vi "Execute Menu Action.vi"(8 "error in":errorcluster, 10 "Item Tag":string, 11 "Peer Review in":refnum<class "Peer Review.lvclass">) -> (0 "error out":errorcluster, 3 "Peer Review out":refnum<class "Peer Review.lvclass">)   [LabVIEW 2020, in "Peer Review.lvclass"]
uses:
  Peer Review.lvclass
  Peer Review.lvclass/Peer Review.ctl
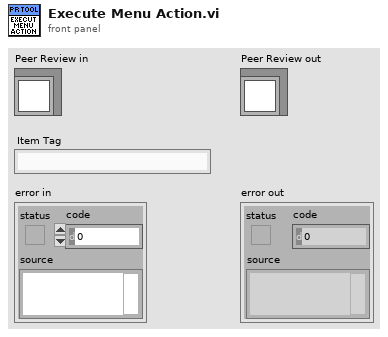
[diagram p1: front panel]
types:
  T1 = typedef "Peer Review.lvclass/File Info.ctl" = cluster{"File ID":i32, "Commit ID":i32, "Reviewed Hash":string, "Relative Path":string, "File Path":path, "File Checksum":string, "State":T2, "FP Changes":i32, "BD Changes":i32, "FP Bounds Error":dbl, "BD Bounds Error":dbl, "Lines Added":i32, "Lines Removed":i32, "Analysis Passes":i32, "Analysis Fails":i32, "Attribute Changes":i32, "Reentrancy State":string, "Cyclomatic Complexity":i32, "Node Count":i32, "Revision Number":u32, "LabVIEW Version":string, "Description":string, "Master Path":path, "Master Checksum":string, "VI Type":T3, "LabVIEW File":bool, "Review Complete":bool, "File Ref":refnum<vi>, "Master Revision":u32}
  T2 = typedef "Peer Review.lvclass/File State.ctl" = enum16{"Interrogation Needed", "Modified", "Deleted", "Added", "Matches Previous", "No Changes", "Moved", "Empty File"}
  T3 = typedef "Peer Review.lvclass/VI Type.ctl" = enum32{"invalid VI type", "Standard VI", "Control VI", "Global VI", "Polymorphic VI", "Configuration VI", "SubSystem", "Facade VI", "Method VI", "Statechart Diagram VI"}
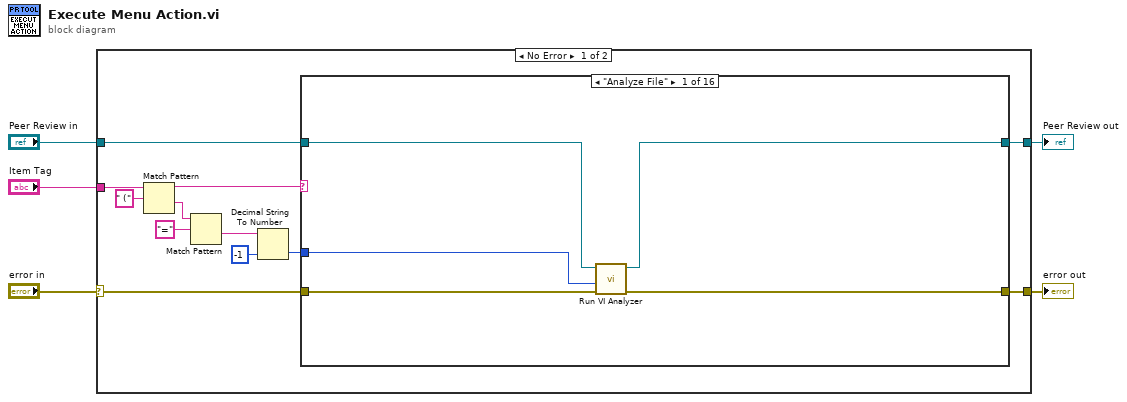
[diagram p0: block diagram]
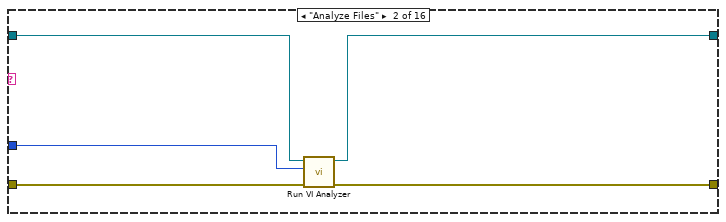
[diagram p2: hidden frame]
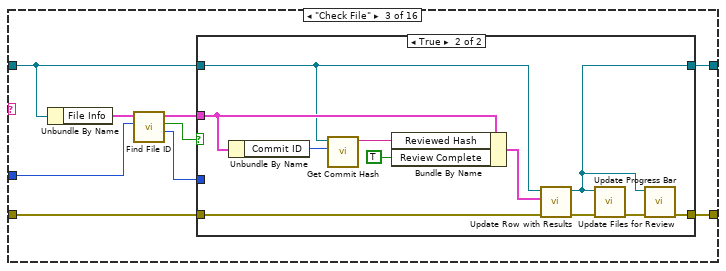
[diagram p3: hidden frame]
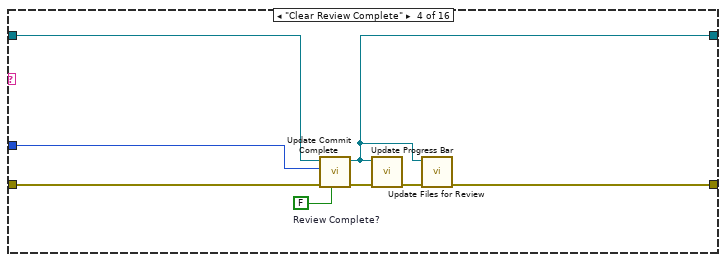
[diagram p5: hidden frame]
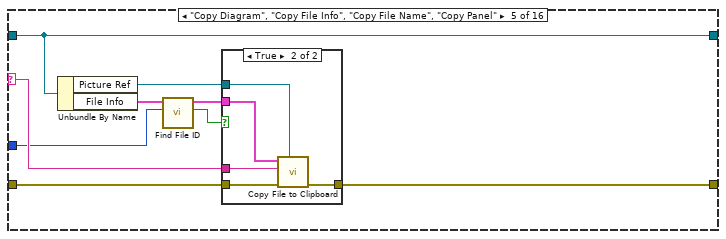
[diagram p6: hidden frame]
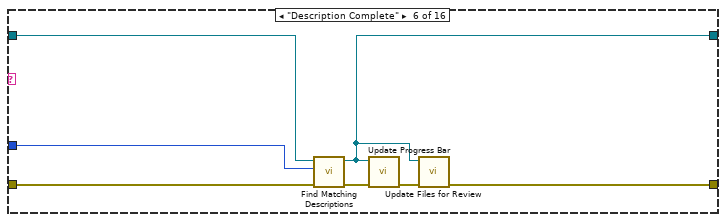
[diagram p8: hidden frame]
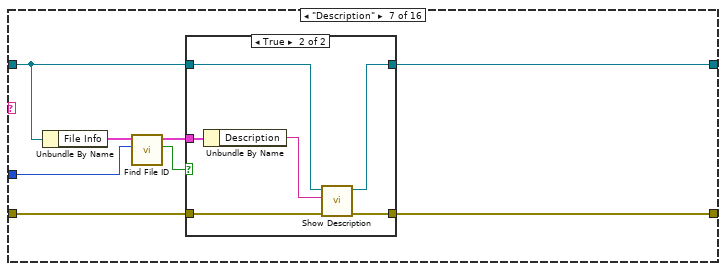
[diagram p9: hidden frame]
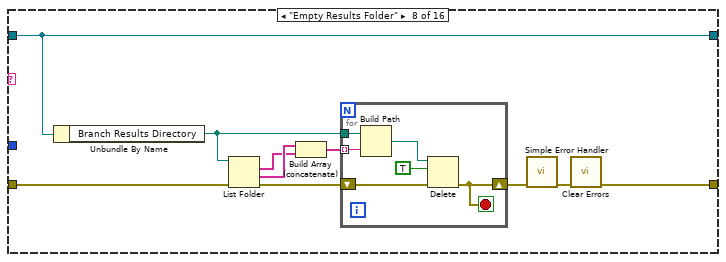
[diagram p11: hidden frame]
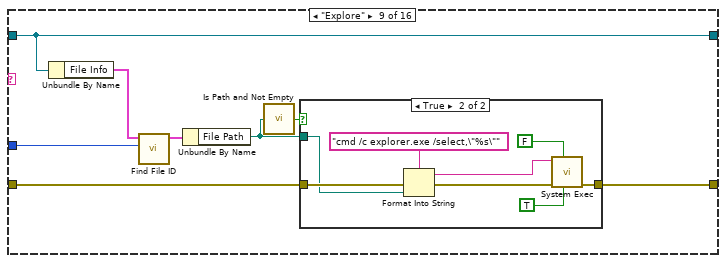
[diagram p12: hidden frame]
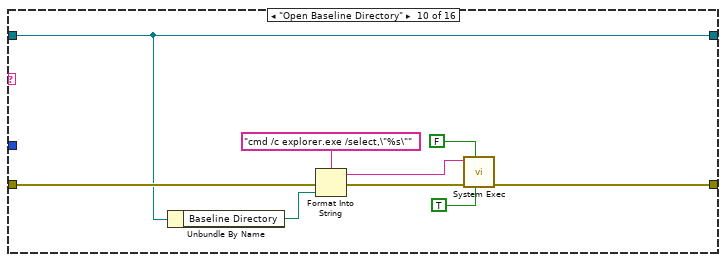
[diagram p14: hidden frame]
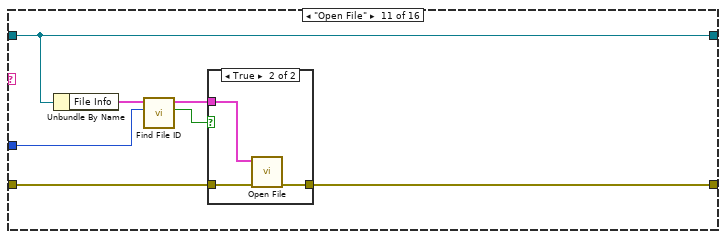
[diagram p15: hidden frame]
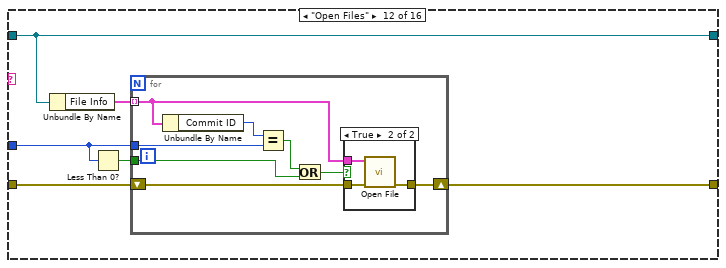
[diagram p17: hidden frame]
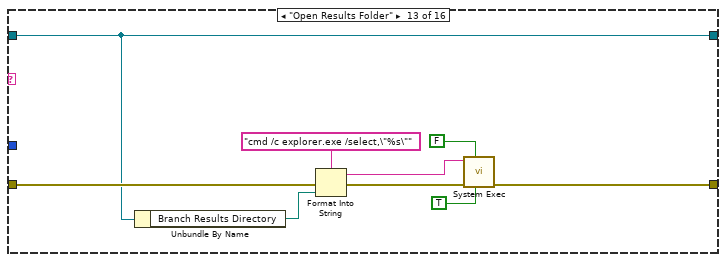
[diagram p19: hidden frame]
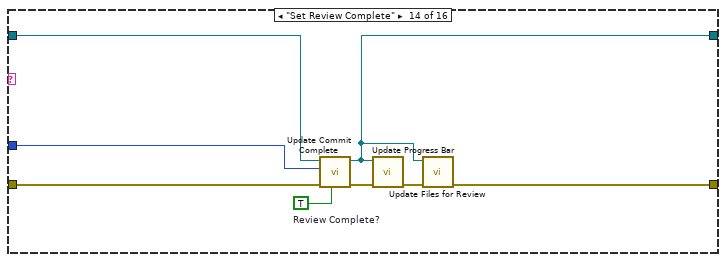
[diagram p20: hidden frame]
diagram:
  n1 = case shown="No Error" "error in" {
    selector: "error in" -> [w9 w207]
    tunnel: "Item Tag" -> [w17 _]
    tunnel: [w8 w207] -> w3
    tunnel: "Peer Review in" -> [w6 w208]
    tunnel: [w7 w208] -> w1
    frame No Error {
      n2 = Match Pattern(string=w17, regular expression=" (") -> (before substring=w15:string, after substring=w14:string)  [unwired: 1 in, 2 out]
      n3 = Match Pattern(string=w14, regular expression="=") -> (after substring=w12:string)  [unwired: 1 in, 3 out]
      n4 = Decimal String To Number(string=w12, default (0L)=-1 ("default (0 I32)")) -> (number=w10:i32)  [unwired: 1 in, 1 out]
      n5 = case shown="\"Analyze File\"" w15 {
        selector: w15 -> [_ _ _ _ w64 _ _ _ _ _ _ _ _ _ _ _]
        tunnel: w10 -> [w18 w26 w36 w55 w61 w77 w82 _ w115 _ w140 w150 _ w181 w192 _]
        tunnel: w6 -> [w20 w24 w33 w56 w63 w78 w85 w105 w117 w131 w144 w151 w169 w182 w189 w205]
        tunnel: w9 -> [w22 w27 w30 w57 w66 w79 w87 w97 w119 w133 w143 w153 w171 w183 w186 w206]
        tunnel: [w21 w25 w29 w51 w65 w74 w86 w103 w118 w132 w142 w152 w170 w177 w185 w206] -> w8
        tunnel: [w19 w23 w34 w50 w63 w73 w84 w105 w117 w131 w144 w151 w169 w176 w190 w205] -> w7
        frame "Analyze File" {
          n6 = call "Run VI Analyzer.vi"("error in"=w22, "File ID"=w18, "Peer Review in"=w20) -> ("error out"=w21:errorcluster, "Peer Review out"=w19:refnum<class "Peer Review.lvclass">)  [unwired: 7 in]
        }
        frame "Analyze Files" {
          n7 = call "Run VI Analyzer.vi"("error in"=w27, "Commit ID"=w26, "Peer Review in"=w24) -> ("error out"=w25:errorcluster, "Peer Review out"=w23:refnum<class "Peer Review.lvclass">)  [unwired: 7 in]
        }
        frame "Check File" {
          n8 = Unbundle By Name(w33) -> ("File Info"=w31:T1[])
          n9 = call "Find File ID.vi"("File ID"=w36, "File List"=w31) -> ("Array Index"=w28:i32, "Found?"=w35:bool, "File Info"=w32:T1)  [unwired: 7 in]
          n10 = case shown="True" w35 {
            tunnel: [w38 w39] -> w34
            tunnel: w33 -> [w38 w45]
            tunnel: w32 -> [_ w46]
            tunnel: w30 -> [w37 w48]
            tunnel: [w37 w40] -> w29
            tunnel: w28 -> [_ _]
            frame False {
            }
            frame True {
              n11 = Unbundle By Name(w46) -> ("Commit ID"=w44:i32)
              n12 = call "Get Commit Hash.vi"("Commit ID"=w44, "Peer Review"=w45) -> ("Hash"=w43:string)  [unwired: 9 in]
              n13 = Bundle By Name(cluster=w46, "Reviewed Hash"=w43, "Review Complete"=TRUE ("Review Complete?")) -> (w47:T1)
              n14 = call "Update Row with Results.vi"("error in"=w48, "File Info"=w47, "Peer Review in"=w45) -> ("error out"=w41:errorcluster, "Peer Review out"=w39:refnum<class "Peer Review.lvclass">)  [unwired: 7 in]
              n15 = call "Update Progress Bar.vi"("error in"=w41, "Peer Review"=w39) -> ("error out"=w42:errorcluster)  [unwired: 9 in]
              n16 = call "Update Files for Review.vi"("error in"=w42, "Peer Review"=w39) -> ("error out"=w40:errorcluster)  [unwired: 9 in]
            }
          }
        }
        frame "Clear Review Complete" {
          w54 = FALSE  # Review Complete?
          n17 = call "Update Commit Complete.vi"("Review Complete?"=w54, "error in"=w57, "Commit ID"=w55, "Peer Review in"=w56) -> ("error out"=w52:errorcluster, "Peer Review out"=w50:refnum<class "Peer Review.lvclass">)  [unwired: 6 in]
          n18 = call "Update Progress Bar.vi"("error in"=w52, "Peer Review"=w50) -> ("error out"=w53:errorcluster)  [unwired: 9 in]
          n19 = call "Update Files for Review.vi"("error in"=w53, "Peer Review"=w50) -> ("error out"=w51:errorcluster)  [unwired: 9 in]
        }
        frame "Copy Diagram", "Copy File Info", "Copy File Name", "Copy Panel" {
          n20 = Unbundle By Name(w63) -> ("Picture Ref"=w58:refnum<vi>, "File Info"=w62:T1[])
          n21 = call "Find File ID.vi"("File ID"=w61, "File List"=w62) -> ("Found?"=w59:bool, "File Info"=w60:T1)  [unwired: 7 in, 1 out]
          n22 = case shown="True" w59 {
            tunnel: w66 -> [w67 w72]
            tunnel: [w67 w71] -> w65
            tunnel: w60 -> [_ w70]
            tunnel: w64 -> [_ w69]
            tunnel: w58 -> [_ w68]
            frame False {
            }
            frame True {
              n23 = call "Copy File to Clipboard.vi"("Picture Ref"=w68, "error in"=w72, "State"=w69, "File Info"=w70) -> ("error out"=w71:errorcluster)  [unwired: 7 in]
            }
          }
        }
        frame "Description Complete" {
          n24 = call "Find Matching Descriptions.vi"("error in"=w79, "File ID"=w77, "Peer Review in"=w78) -> ("error out"=w75:errorcluster, "Peer Review out"=w73:refnum<class "Peer Review.lvclass">)  [unwired: 7 in]
          n25 = call "Update Progress Bar.vi"("error in"=w75, "Peer Review"=w73) -> ("error out"=w76:errorcluster)  [unwired: 9 in]
          n26 = call "Update Files for Review.vi"("error in"=w76, "Peer Review"=w73) -> ("error out"=w74:errorcluster)  [unwired: 9 in]
        }
        frame "Description" {
          n27 = Unbundle By Name(w85) -> ("File Info"=w83:T1[])
          n28 = call "Find File ID.vi"("File ID"=w82, "File List"=w83) -> ("Found?"=w81:bool, "File Info"=w80:T1)  [unwired: 7 in, 1 out]
          n29 = case shown="True" w81 {
            tunnel: w87 -> [w89 w95]
            tunnel: [w89 w94] -> w86
            tunnel: w85 -> [w88 w93]
            tunnel: [w88 w92] -> w84
            tunnel: w80 -> [_ w91]
            frame False {
            }
            frame True {
              n30 = Unbundle By Name(w91) -> ("Description"=w90:string)
              n31 = call "Show Description.vi"("error in"=w95, "Description"=w90, "Peer Review in"=w93) -> ("error out"=w94:errorcluster, "Peer Review out"=w92:refnum<class "Peer Review.lvclass">)  [unwired: 7 in]
            }
          }
        }
        frame "Empty Results Folder" {
          n32 = Unbundle By Name(w105) -> ("Branch Results Directory"=w96:path)
          n33 = List Folder(path=w96, error in=w97) -> (filenames=w101:string[], folder names=w102:string[], error out=w99:errorcluster)  [unwired: 2 in, 1 out]
          n34 = Build Array (concatenate)(w102, w101) -> (w100:string[])
          n35 = for {
            tunnel: w96 -> [w111]
            tunnel: w100 -> [w110] mode=indexing
            shift-right: [w106] -> w98
            shift-left: w99 -> [w108]
            stop <- w106 stop-if-true
            n36 = Build Path(base path=w111, name or relative path=w110) -> (appended path=w109:path)
            n37 = Delete(path (use dialog)=w109, entire hierarchy (F)=TRUE, error in=w108) -> (error out=w106:errorcluster)  [unwired: 2 in, 2 out]
          }
          n38 = call <vilib>:"Simple Error Handler.vi"("error in (no error)"=w98) -> ("error out"=w104:errorcluster)  [unwired: 4 in, 4 out]
          n39 = call <vilib>:"Clear Errors.vi"("error in (no error)"=w104) -> ("error out"=w103:errorcluster)  [unwired: 5 in, 1 out]
        }
        frame "Explore" {
          n40 = Unbundle By Name(w117) -> ("File Info"=w116:T1[])
          n41 = call "Find File ID.vi"("File ID"=w115, "File List"=w116) -> ("File Info"=w114:T1)  [unwired: 7 in, 2 out]
          n42 = Unbundle By Name(w114) -> ("File Path"=w113:path)
          n43 = call <vilib>:"Is Path and Not Empty.vi"("path"=w113) -> ("Is Path and Not Empty?"=w112:bool)  [unwired: 4 in]
          n44 = case shown="True" w112 {
            tunnel: w119 -> [w120 w124]
            tunnel: [w120 w123] -> w118
            tunnel: w113 -> [_ w121]
            frame False {
            }
            frame True {
              n45 = Format Into String(format string="cmd /c explorer.exe /select,\"%s\"" ("string"), error in=w124, w121) -> (resulting string=w125:string, error out=w127:errorcluster)  [unwired: 1 in]
              n46 = call <vilib>:"System Exec.vi"("run minimized? (F)"=TRUE, "wait until completion? (T)"=FALSE, "error in (no error)"=w127, "command line"=w125) -> ("error out"=w123:errorcluster)  [unwired: 4 in, 3 out]
            }
          }
        }
        frame "Open Baseline Directory" {
          n47 = Unbundle By Name(w131) -> ("Baseline Directory"=w130:path)
          n48 = Format Into String(format string="cmd /c explorer.exe /select,\"%s\"" ("string"), error in=w133, w130) -> (resulting string=w134:string, error out=w136:errorcluster)  [unwired: 1 in]
          n49 = call <vilib>:"System Exec.vi"("run minimized? (F)"=TRUE, "wait until completion? (T)"=FALSE, "error in (no error)"=w136, "command line"=w134) -> ("error out"=w132:errorcluster)  [unwired: 4 in, 3 out]
        }
        frame "Open File" {
          n50 = Unbundle By Name(w144) -> ("File Info"=w141:T1[])
          n51 = call "Find File ID.vi"("File ID"=w140, "File List"=w141) -> ("Found?"=w139:bool, "File Info"=w138:T1)  [unwired: 7 in, 1 out]
          n52 = case shown="True" w139 {
            tunnel: w143 -> [w145 w148]
            tunnel: [w145 w147] -> w142
            tunnel: w138 -> [_ w146]
            frame False {
            }
            frame True {
              n53 = call "Open File.vi"("error in"=w148, "File Info"=w146) -> ("error out"=w147:errorcluster)  [unwired: 9 in]
            }
          }
        }
        frame "Open Files" {
          n54 = Unbundle By Name(w151) -> ("File Info"=w154:T1[])
          n55 = Less Than 0?(x=w150) -> (x < 0?=w149:bool)
          n56 = for {
            tunnel: w154 -> [w158] mode=indexing
            shift-right: [w159] -> w152
            shift-left: w153 -> [w160]
            tunnel: w150 -> [w162]
            tunnel: w149 -> [w157]
            n57 = Unbundle By Name(w158) -> ("Commit ID"=w161:i32)
            n58 = Equal?(x=w161, y=w162) -> (x = y?=w156:bool)
            n59 = Or(x=w156, y=w157) -> (x .or. y?=w155:bool)
            n60 = case shown="True" w155 {
              tunnel: w160 -> [w163 w166]
              tunnel: [w163 w165] -> w159
              tunnel: w158 -> [_ w164]
              frame False {
              }
              frame True {
                n61 = call "Open File.vi"("error in"=w166, "File Info"=w164) -> ("error out"=w165:errorcluster)  [unwired: 9 in]
              }
            }
          }
        }
        frame "Open Results Folder" {
          n62 = Unbundle By Name(w169) -> ("Branch Results Directory"=w168:path)
          n63 = Format Into String(format string="cmd /c explorer.exe /select,\"%s\"" ("string"), error in=w171, w168) -> (resulting string=w172:string, error out=w174:errorcluster)  [unwired: 1 in]
          n64 = call <vilib>:"System Exec.vi"("run minimized? (F)"=TRUE, "wait until completion? (T)"=FALSE, "error in (no error)"=w174, "command line"=w172) -> ("error out"=w170:errorcluster)  [unwired: 4 in, 3 out]
        }
        frame "Set Review Complete" {
          w180 = TRUE  # Review Complete?
          n65 = call "Update Commit Complete.vi"("Review Complete?"=w180, "error in"=w183, "Commit ID"=w181, "Peer Review in"=w182) -> ("error out"=w178:errorcluster, "Peer Review out"=w176:refnum<class "Peer Review.lvclass">)  [unwired: 6 in]
          n66 = call "Update Progress Bar.vi"("error in"=w178, "Peer Review"=w176) -> ("error out"=w179:errorcluster)  [unwired: 9 in]
          n67 = call "Update Files for Review.vi"("error in"=w179, "Peer Review"=w176) -> ("error out"=w177:errorcluster)  [unwired: 9 in]
        }
        frame "Uncheck File" {
          n68 = Unbundle By Name(w189) -> ("File Info"=w187:T1[])
          n69 = call "Find File ID.vi"("File ID"=w192, "File List"=w187) -> ("Array Index"=w184:i32, "Found?"=w191:bool, "File Info"=w188:T1)  [unwired: 7 in]
          n70 = case shown="True" w191 {
            tunnel: [w194 w195] -> w190
            tunnel: w189 -> [w194 w200]
            tunnel: w188 -> [_ w204]
            tunnel: w186 -> [w193 w202]
            tunnel: [w193 w196] -> w185
            tunnel: w184 -> [_ _]
            frame False {
            }
            frame True {
              n71 = Bundle By Name(cluster=w204, "Reviewed Hash"="", "Review Complete"=FALSE ("Review Complete?")) -> (w201:T1)
              n72 = call "Update Row with Results.vi"("error in"=w202, "File Info"=w201, "Peer Review in"=w200) -> ("error out"=w197:errorcluster, "Peer Review out"=w195:refnum<class "Peer Review.lvclass">)  [unwired: 7 in]
              n73 = call "Update Progress Bar.vi"("error in"=w197, "Peer Review"=w195) -> ("error out"=w198:errorcluster)  [unwired: 9 in]
              n74 = call "Update Files for Review.vi"("error in"=w198, "Peer Review"=w195) -> ("error out"=w196:errorcluster)  [unwired: 9 in]
            }
          }
        }
        frame Default {
        }
      }
    }
    frame Error {
    }
  }
  "error out" <- w3
  "Peer Review out" <- w1
